vi "Node - Byte Buffer Read - Runtime.vi"(8 "error in (no error)":errorcluster, 11 "Node Data In":T1) -> (0 "error out":errorcluster, 1 "Channel Data Out":dbl[](array[numeric]), 3 "Node Data Out":T1)   [LabVIEW 2016, in "PXImc Router.lvlib"]
uses:
  PXImc Router.lvlib
  Controls/Node Data.ctl
  <vilib>/NI Veristand/VeriStand Data/Byte Buffer/Byte Buffer.lvclass
  Controls/Node/Node - PXImc Parameters.ctl
  Controls/Node/Transfer Data.ctl
  Controls/Node/Node Ch Properties.ctl
  Controls/Data Type.ctl
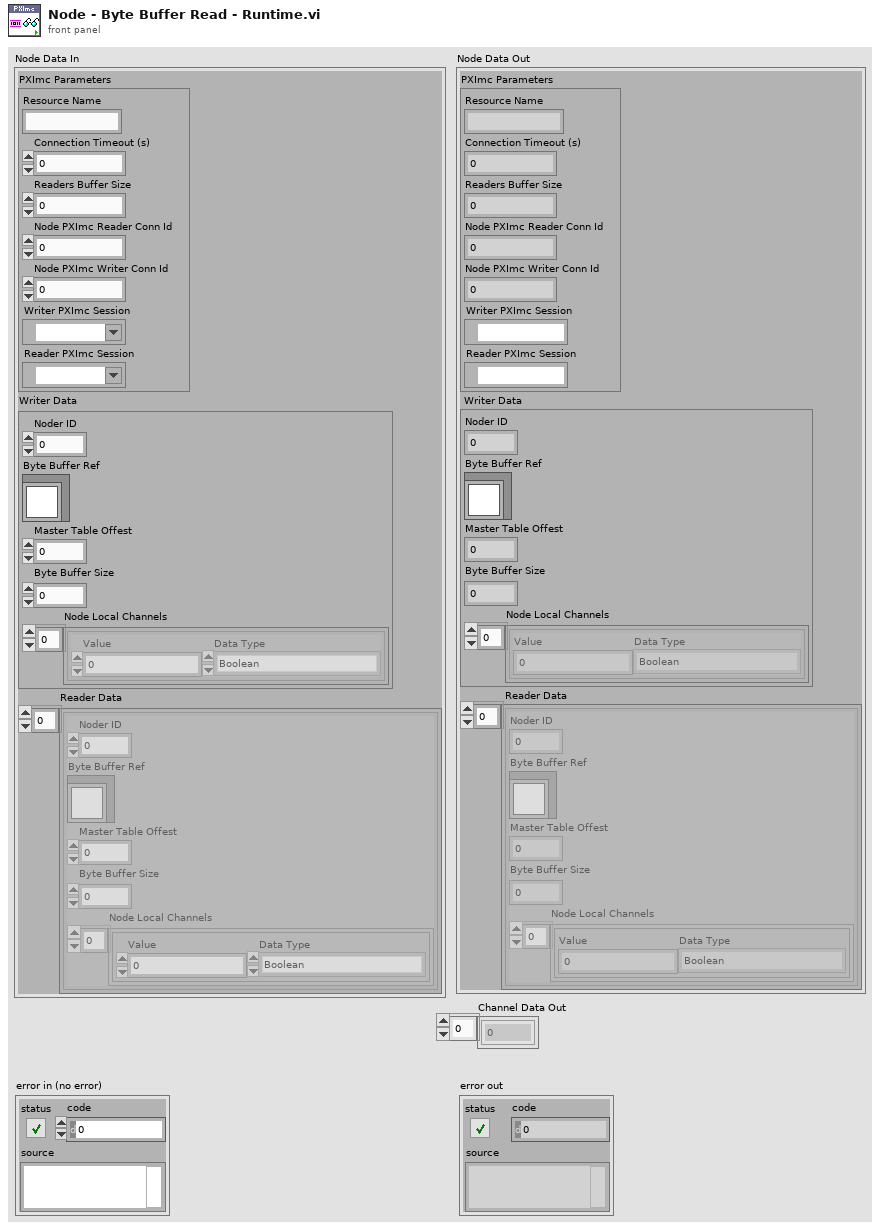
[diagram p1: front panel]
types:
  T1 = typedef "PXImc Router.lvlib/Node Data.ctl" = cluster{"PXImc Parameters":T2, "Writer Data":T3, "Reader Data":T3[]}
  T2 = typedef "PXImc Router.lvlib/Node - PXImc Parameters.ctl" = cluster{"Resource Name":string, "Connection Timeout (s)":dbl, "Readers Buffer Size":u64, "Node PXImc Reader Conn Id":u16, "Node PXImc Writer Conn Id":u16, "Writer PXImc Session":refnum<k21>, "Reader PXImc Session":refnum<k21>}
  T3 = typedef "PXImc Router.lvlib/Transfer Data.ctl" = cluster{"Noder ID":u32, "Byte Buffer Ref":refnum<class "Byte Buffer.lvclass">, "Master Table Offest":u32, "Byte Buffer Size":u32, "Node Local Channels":T4[]}
  T4 = typedef "PXImc Router.lvlib/Node Ch Properties.ctl" = cluster{"Value":dbl, "Data Type":T5}
  T5 = typedef "PXImc Router.lvlib/Data Type.ctl" = enum16{"Boolean", "SGL", "DBL", "I8", "I16", "I32", "I64", "U8", "U16", "U32", "U64"}
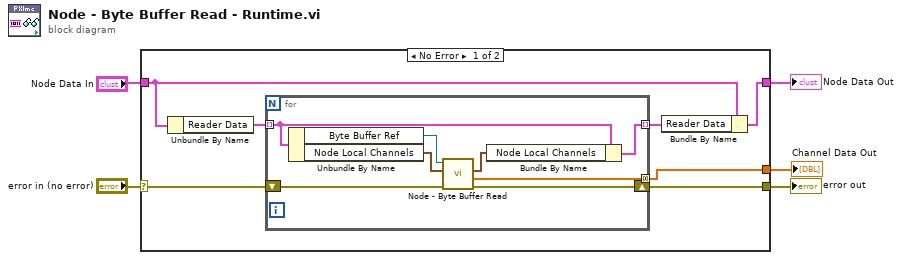
[diagram p0: block diagram]
diagram:
  n1 = case shown="No Error" "error in (no error)" {
    selector: "error in (no error)" -> [w10 w21]
    tunnel: "Node Data In" -> [w12 w22]
    tunnel: [w11 w22] -> w4
    tunnel: [w9 w21] -> w2
    tunnel: [w6 _] -> w1
    frame No Error {
      n2 = Unbundle By Name(w12) -> ("Reader Data"=w8:T3[])
      n3 = for {
        shift-right: [w19] -> w9
        shift-left: w10 -> [w20]
        tunnel: w8 -> [w17] mode=indexing
        tunnel: [w15] -> w7 mode=indexing
        tunnel: [w13] -> w6 mode=concatenating
        n4 = Unbundle By Name(w17) -> ("Byte Buffer Ref"=w16:refnum<class "Byte Buffer.lvclass">, "Node Local Channels"=w18:T4[])
        n5 = call "Node - Byte Buffer Read.vi"("error in (no error)"=w20, "Node Local Channels In"=w18, "Byte Buffer In"=w16) -> ("error out"=w19:errorcluster, "Channel Data Out"=w13:dbl[], "Node Local Channels Out"=w14:T4[])  [unwired: 5 in, 1 out]
        n6 = Bundle By Name(cluster=w17, "Node Local Channels"=w14) -> (w15:T3)
      }
      n7 = Bundle By Name(cluster=w12, "Reader Data"=w7) -> (w11:T1)
    }
    frame Error {
    }
  }
  "error out" <- w2
  "Node Data Out" <- w4
  "Channel Data Out" <- w1
